vi "Vision Code_2.vi"(0 "Image In":T1, 1 "Image Dst":T1, 2 "Final Image Output":T1, 7 "error in":errorcluster) -> (20 "Image Out":T1, 21 "Output Image":T1(plugin-control), 27 "error out":errorcluster)   [LabVIEW 2014]
doc: "Creates, edits, and runs vision algorithms using NI Vision Assistant.\n\nWhen you place this Express VI on the block diagram, NI Vision Assistant launches. Create an algorithm using the Vision Assistant processing functions. After you create an algorithm, you can select the controls and indicators that you want to be able to programmatically set in LabVIEW. Double-click the Vision Assistant Express VI to edit the algorithm."
uses:
  <vilib>/vision/Image Controls.llb/IMAQ Image.ctl
  <vilib>/vision/NI_Vision_Development_Module.lvlib
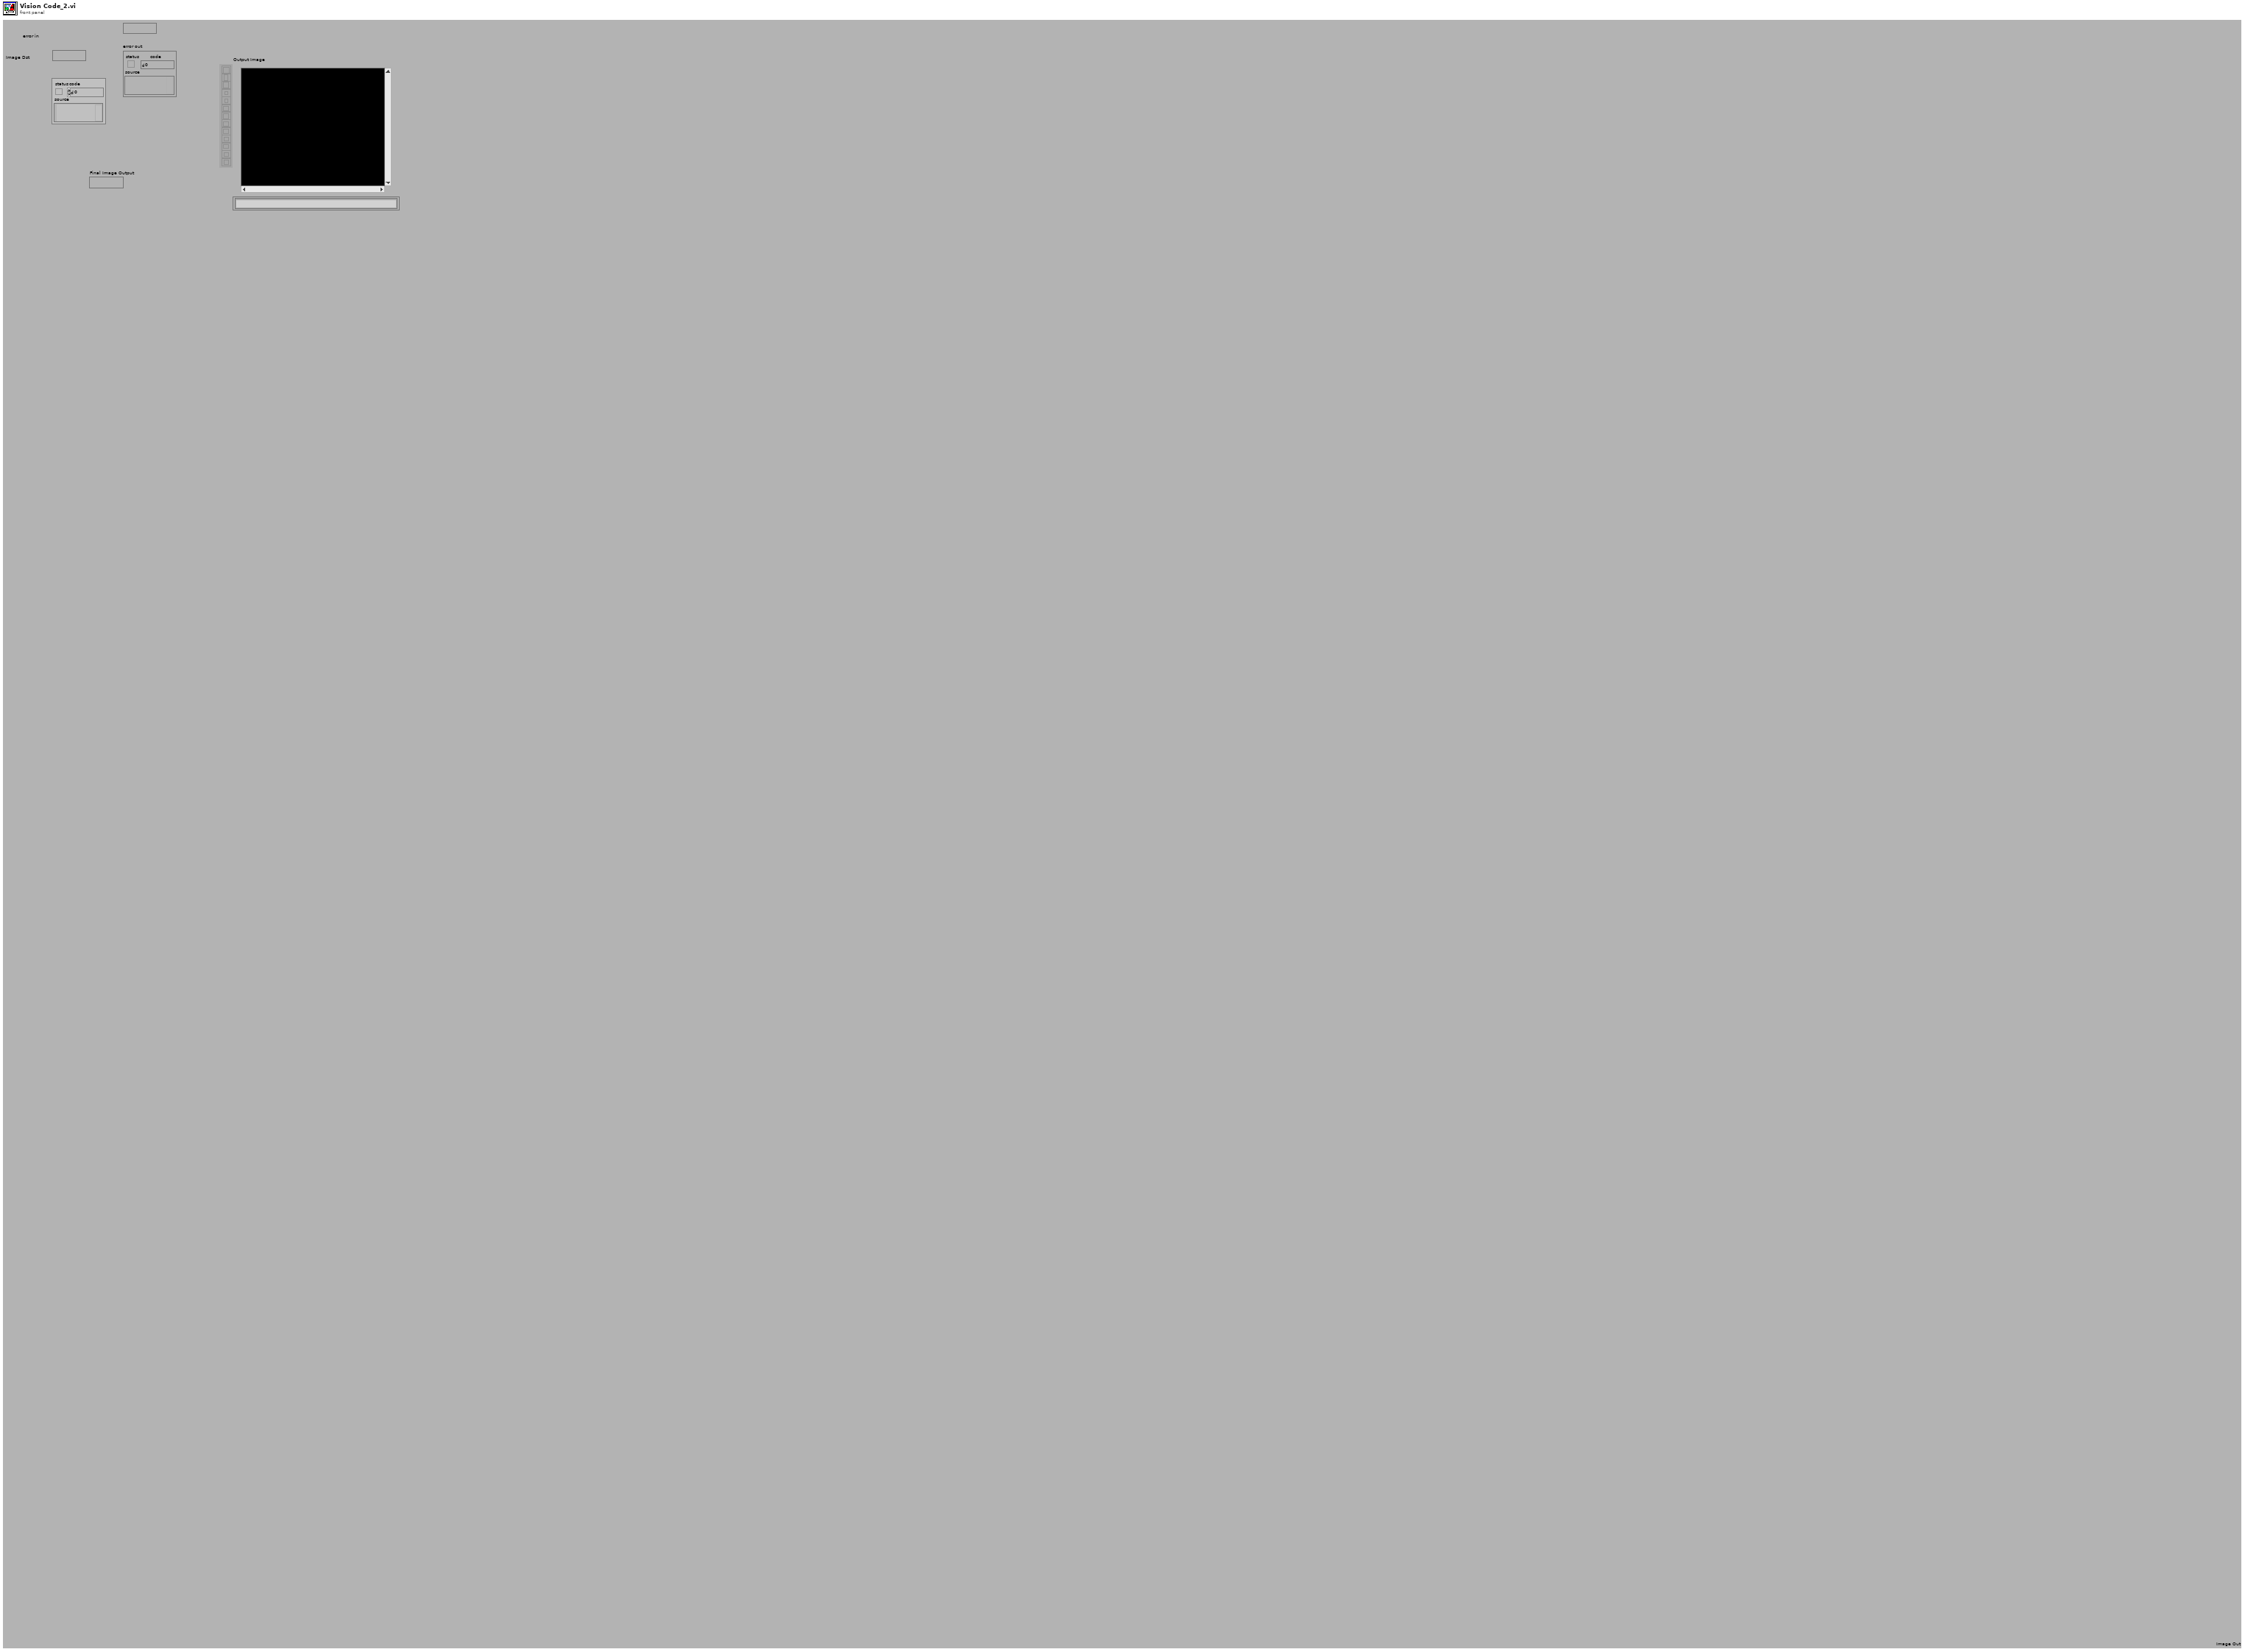
[diagram p1: front panel]
types:
  T1 = typedef "IMAQ Image.ctl" = refnum<image>
  T2 = cluster{"Sigma":sgl, "HThresh":sgl, "LThres":sgl, "WindowSize":i32}
  T3 = enum32{"AutoM", "Close", "Dilate", "Erode", "Gradient", "Gradient out", "Gradient in", "Hit miss", "Open", "PClose", "POpen", "Thick", "Thin"}
  T4 = typedef "Image Type" = u32
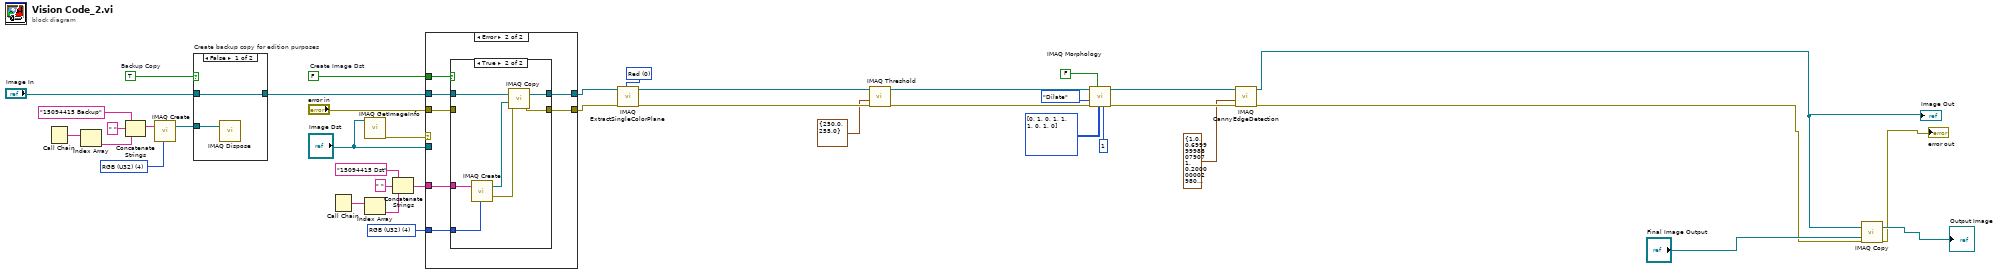
[diagram p0: block diagram]
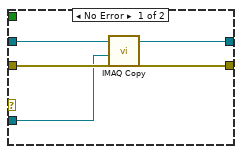
[diagram p2: hidden frame]
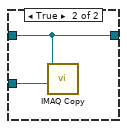
[diagram p4: hidden frame]
diagram:
  w17 = 0 items=["Red", "Green", "Blue", "Hue", "Saturation", "Luminance", "Value", "Intensity"] ("Color Plane")
  w21 = T4 4 items=["Grayscale (U8)", "Grayscale (I16)", "Grayscale (SGL)", "Complex (CSG)", "RGB (U32)", "HSL (U32)", "RGB (U64)", "Grayscale (U16)"] ("Image Dst Type")
  w22 = T4 4 items=["Grayscale (U8)", "Grayscale (I16)", "Grayscale (SGL)", "Complex (CSG)", "RGB (U32)", "HSL (U32)", "RGB (U64)", "Grayscale (U16)"] ("Image Type")
  w40 = TRUE  # Backup Copy
  w34 = FALSE  # Create Image Dst
  n1 = Call Chain() -> (call chain=w28:string[])
  n2 = Index Array(array=w28) -> (element=w27:string)  [unwired: 1 in]
  n3 = Concatenate Strings("15094415 Backup" ("Backup Image Name"), " ", w27) -> (w24:string)
  n4 = call "IMAQ Create"("Image Name"=w24, "Image Type"=w22) -> ("New Image"=w23:T1)  [unwired: 2 in, 2 out]
  n5 = case "Create backup copy for edition purposes" shown="False" w40 {
    tunnel: [w42 w44] -> w36
    tunnel: "Image In" -> [w42 w44]
    tunnel: w23 -> [w41 w43]
    frame False {
      n6 = call "IMAQ Dispose"("Image"=w41) -> ()  [unwired: 2 in, 4 out]
    }
    frame True {
      n7 = call "IMAQ Copy"("Image Dst"=w43, "Image Src"=w44) -> ()  [unwired: 1 in, 5 out]
    }
  }
  n8 = Call Chain() -> (call chain=w33:string[])
  n9 = call "IMAQ GetImageInfo"("Image"="Image Dst") -> ("error out"=w38:errorcluster)  [unwired: 1 in, 9 out]
  n10 = Index Array(array=w33) -> (element=w31:string)  [unwired: 1 in]
  n11 = Concatenate Strings("15094415 Dst" ("Image Dst Name"), " ", w31) -> (w29:string)
  n12 = case shown="Error" w38 {
    tunnel: [w49 w53] -> w6
    tunnel: [w48 w52] -> w7
    tunnel: w36 -> [w47 w54]
    tunnel: "error in" -> [w46 w50]
    tunnel: "Image Dst" -> [w45 _]
    tunnel: w29 -> [_ w56]
    tunnel: w21 -> [_ w55]
    tunnel: w34 -> [_ w51]
    frame No Error {
      n13 = call "IMAQ Copy"("error in (no error)"=w46, "Image Dst"=w45, "Image Src"=w47) -> ("error out"=w48:errorcluster, "Image Dst Out"=w49:T1)  [unwired: 3 out]
    }
    frame Error {
      n14 = case shown="True" w51 {
        tunnel: w56 -> [_ w65]
        tunnel: w55 -> [_ w64]
        tunnel: w54 -> [w58 w62]
        tunnel: [w58 w61] -> w53
        tunnel: [w57 w60] -> w52
        tunnel: w50 -> [w57 _]
        frame False {
        }
        frame True {
          n15 = call "IMAQ Create"("Image Name"=w65, "Image Type"=w64) -> ("New Image"=w63:T1, "error out"=w59:errorcluster)  [unwired: 2 in, 1 out]
          n16 = call "IMAQ Copy"("error in (no error)"=w59, "Image Dst"=w63, "Image Src"=w62) -> ("error out"=w60:errorcluster, "Image Dst Out"=w61:T1)  [unwired: 3 out]
        }
      }
    }
  }
  n17 = call "IMAQ ExtractSingleColorPlane"("Color Plane"=w17, "error in (no error)"=w7, "Image Src"=w6) -> ("error out"=w16:errorcluster, "Image Dst Out"=w14:T1)  [unwired: 1 in, 6 out]
  n18 = call "IMAQ Threshold"("error in (no error)"=w16, "Range"=cluster{"Lower value":sgl, "Upper value":sgl} {"Lower value"=250.0, "Upper value"=255.0}, "Image Src"=w14) -> ("error out"=w13:errorcluster, "Image Dst Out"=w8:T1)  [unwired: 3 in, 4 out]
  n19 = call "IMAQ Morphology"("Number of iterations (1)"=1, "Structuring Element"=i32[][] [[0, 1, 0], [1, 1, 1], [0, 1, 0]], "Square/Hexa (Square)"=FALSE, "error in (no error)"=w13, "Operation"=T3."Dilate", "Image Src"=w8) -> ("error out"=w4:errorcluster, "Image Dst Out"=w5:T1)  [unwired: 1 in, 3 out]
  n20 = call "IMAQ CannyEdgeDetection"("Image Src"=w5, "Filter Parameters"=T2 {"Sigma"=1.0, "HThresh"=0.7, "LThres"=0.2, "WindowSize"=9}, "error in (no error)"=w4) -> ("Image Dst Out"=w2:T1, "error out"=w3:errorcluster)  [unwired: 5 in]
  "Image Out" <- w2
  n21 = call "IMAQ Copy"("error in (no error)"=w3, "Image Dst"="Final Image Output", "Image Src"=w2) -> ("error out"=→"error out":errorcluster, "Image Dst Out"=→"Output Image":T1)  [unwired: 3 out]
